vi "Stop.vi"(8 "error in (no error)":errorcluster, 11 "CAN_Logic in":refnum<class "CAN_Logic.lvclass">) -> (0 "error out":errorcluster, 3 "CAN_Logic out":refnum<class "CAN_Logic.lvclass">)   [LabVIEW 2021, in "CAN_Logic.lvclass"]
uses:
  CAN_Logic.lvclass
  CAN_Logic.lvclass/CAN_Logic.ctl
  <vilib>/xnet/xnet.llb/XNET Wait (Transmit Complete).vi
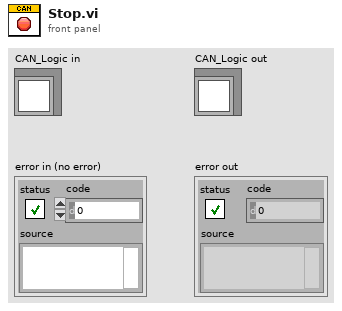
[diagram p1: front panel]
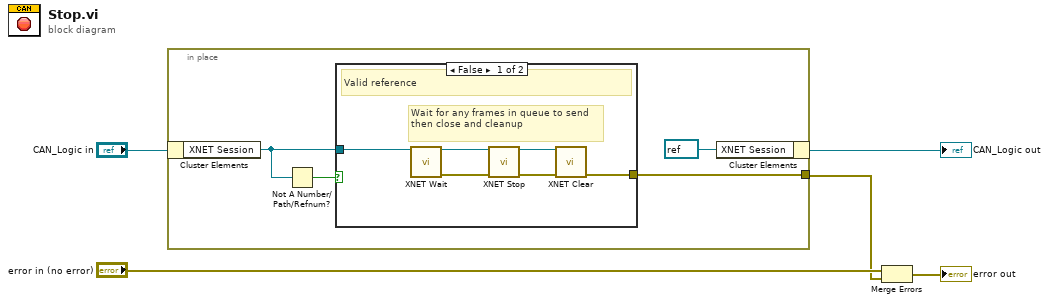
[diagram p0: block diagram]
diagram:
  n1 = in-place {
    in-place-border: [w6] -> w2
    n2 = in-place-cluster #1("CAN_Logic in") -> ("XNET Session"=w8:refnum<k21>)
    n3 = Not A Number/Path/Refnum?(number/path/refnum=w8) -> (NaN/Path/Refnum?=w9:bool)
    n4 = case shown="False" w9 {
      tunnel: w8 -> [w15 _]
      tunnel: [w10 _] -> w6
      frame False {
        # "Wait for any frames in queue to send then close and cleanup"
        # "Valid reference"
        n5 = call-poly <vilib>:"XNET Wait.vi"("session in"=w15) -> ("session out"=w14:refnum<k21>, "error out"=w13:errorcluster)  [unwired: 13 in]
        n6 = call <vilib>:"XNET Stop.vi"("session in"=w14, "error in (no error)"=w13) -> ("session out"=w12:refnum<k21>, "error out"=w11:errorcluster)  [unwired: 12 in]
        n7 = call <vilib>:"XNET Clear.vi"("session in"=w12, "error in (no error)"=w11) -> ("error out"=w10:errorcluster)  [unwired: 13 in]
      }
      frame True {
        # "Not valid reference"
      }
    }
    n8 = in-place-cluster #1("XNET Session"=refnum<k21> refnum) -> (→"CAN_Logic out":refnum<class "CAN_Logic.lvclass">)
  }
  n9 = Merge Errors("error in (no error)", w2) -> (→"error out":errorcluster)
